vi "DZIELENIE_Z_RESZTA.vi"() -> ()   [LabVIEW 2018]
panel:
  out "reszta":dbl
  out "iloraz":dbl
  in  "dzielnik(ró¿ny od 0)":dbl
  in  "dzielna":dbl
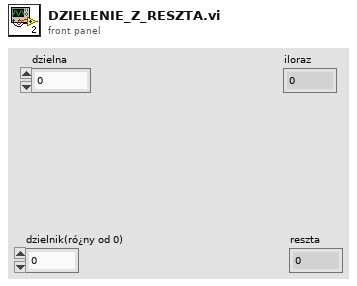
[diagram p1: front panel]
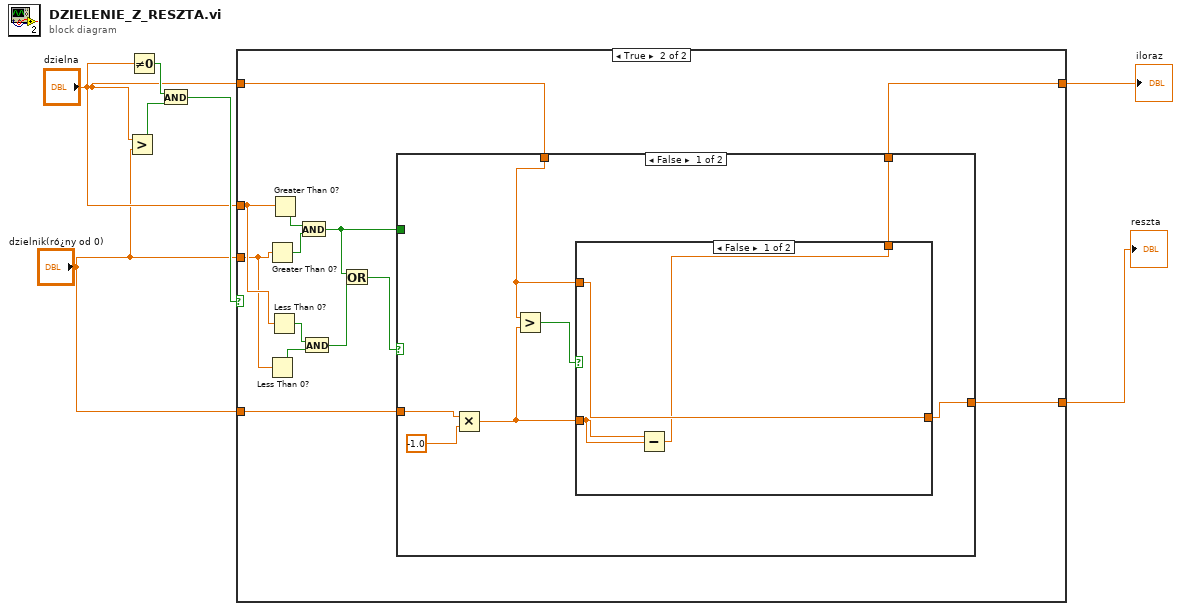
[diagram p0: block diagram]
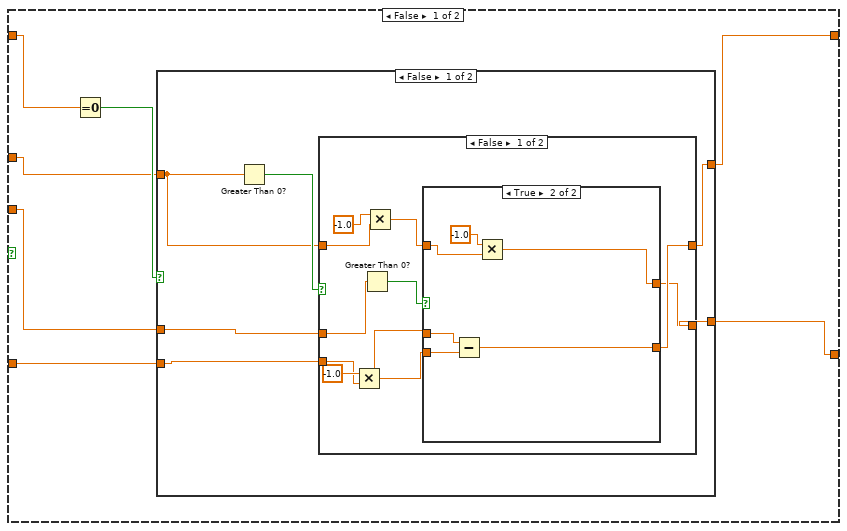
[diagram p2: hidden frame]
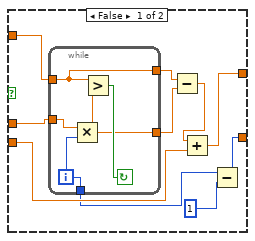
[diagram p3: hidden frame]
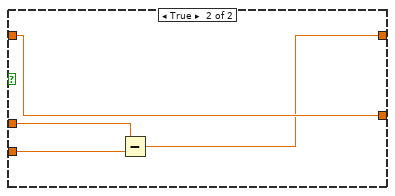
[diagram p4: hidden frame]
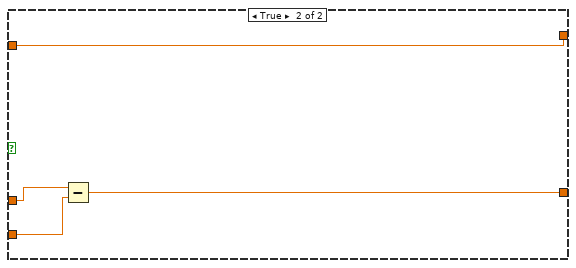
[diagram p5: hidden frame]
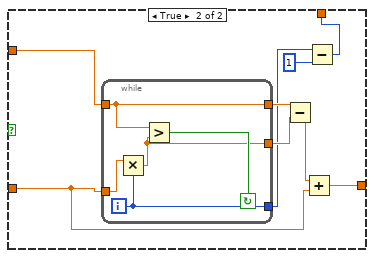
[diagram p6: hidden frame]
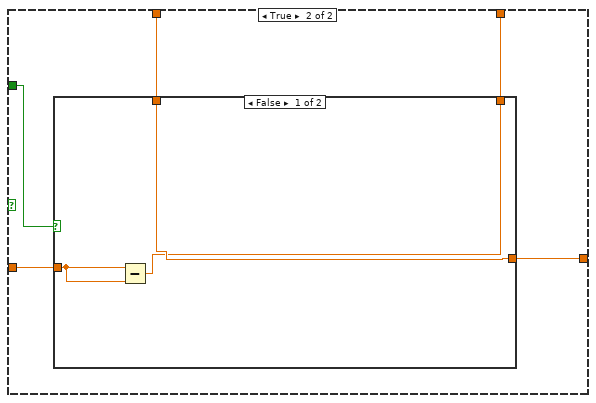
[diagram p7: hidden frame]
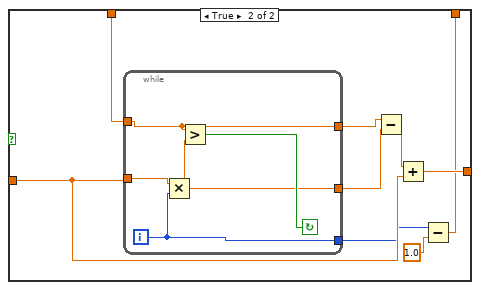
[diagram p8: hidden frame]
diagram:
  n1 = Greater?(x="dzielna", y="dzielnik(ró¿ny od 0)") -> (0:w6:bool)
  n2 = Not Equal To 0?(x="dzielna") -> (x != 0?=w7:bool)
  n3 = And(x=w7, y=w6) -> (x .and. y?=w5:bool)
  n4 = case shown="True" w5 {
    tunnel: "dzielna" -> [w12 w72]
    tunnel: "dzielnik(ró¿ny od 0)" -> [w11 w71]
    tunnel: "dzielna" -> [w14 w63]
    tunnel: "dzielnik(ró¿ny od 0)" -> [w10 w62]
    tunnel: [w9 w61] -> w2
    tunnel: [w8 w60] -> w1
    frame False {
      n5 = Equal To 0?(x=w14) -> (x = 0?=w13:bool)
      n6 = case shown="False" w13 {
        tunnel: w12 -> [w19 w56]
        tunnel: w11 -> [w16 w59]
        tunnel: w10 -> [w15 w58]
        tunnel: [w17 w57] -> w9
        tunnel: [w18 w56] -> w8
        frame False {
          n7 = Greater Than 0?(x=w19) -> (x > 0?=w20:bool)
          n8 = case shown="False" w20 {
            tunnel: w19 -> [w26 w55]
            tunnel: [w28 w52] -> w18
            tunnel: [w27 w55] -> w17
            tunnel: w16 -> [w29 w54]
            tunnel: w15 -> [w22 w53]
            frame False {
              n9 = Multiply(x=-1.0, y=w22) -> (x*y=w21:dbl)
              n10 = Greater Than 0?(x=w29) -> (x > 0?=w30:bool)
              n11 = Multiply(x=-1.0 ("y"), y=w26) -> (x*y=w24:dbl)
              n12 = case shown="True" w30 {
                tunnel: w21 -> [w40 w51]
                tunnel: w21 -> [w38 w50]
                tunnel: [w34 w49] -> w28
                tunnel: w24 -> [w33 w46]
                tunnel: [w37 w47] -> w27
                frame False {
                  n13 = while {
                    tunnel: w33 -> [w43]
                    tunnel: w40 -> [w45]
                    tunnel: [w43] -> w39
                    tunnel: [w42] -> w32
                    tunnel: [w41] -> w36
                    i -> [w41]
                    stop <- w44 continue-if-true
                    n14 = Multiply(x=w45, y=w41) -> (x*y=w42:dbl)
                    n15 = Greater?(x=w43, y=w42) -> (0:w44:bool)
                  }
                  n16 = Subtract(x=w39, y=w32) -> (x-y=w31:dbl)
                  n17 = Add(x=w31, y=w38) -> (x+y=w37:dbl)
                  n18 = Subtract(x=w36, y=1) -> (x-y=w34:i32)
                }
                frame True {
                  n19 = Subtract(x=w51, y=w50) -> (x-y=w49:dbl)
                  n20 = Multiply(x=-1.0 ("x*y"), y=w46) -> (x*y=w47:dbl)
                }
              }
            }
            frame True {
              n21 = Subtract(x=w54, y=w53) -> (x-y=w52:dbl)
            }
          }
        }
        frame True {
          n22 = Subtract(x=w59, y=w58) -> (x-y=w57:dbl)
        }
      }
    }
    frame True {
      n23 = Greater Than 0?(x=w71) -> (x > 0?=w68:bool)
      n24 = Less Than 0?(x=w71) -> (x < 0?=w67:bool)
      n25 = Less Than 0?(x=w72) -> (x < 0?=w69:bool)
      n26 = Greater Than 0?(x=w72) -> (x > 0?=w70:bool)
      n27 = And(x=w70, y=w68) -> (x .and. y?=w64:bool)
      n28 = And(x=w69, y=w67) -> (x .and. y?=w66:bool)
      n29 = Or(x=w64, y=w66) -> (x .or. y?=w65:bool)
      n30 = case shown="False" w65 {
        tunnel: w64 -> [_ w101]
        tunnel: w63 -> [w76 w100]
        tunnel: w62 -> [w79 w99]
        tunnel: [w74 w98] -> w61
        tunnel: [w73 w97] -> w60
        frame False {
          n31 = Multiply(x=w79, y=-1.0 ("x*y")) -> (x*y=w75:dbl)
          n32 = Greater?(x=w76, y=w75) -> (0:w77:bool)
          n33 = case shown="False" w77 {
            tunnel: w76 -> [w82 w91]
            tunnel: w75 -> [w81 w88]
            tunnel: [w82 w86] -> w74
            tunnel: [w80 w85] -> w73
            frame False {
              n34 = Subtract(x=w81, y=w81) -> (x-y=w80:dbl)
            }
            frame True {
              n35 = while {
                tunnel: w91 -> [w94]
                tunnel: w88 -> [w95]
                tunnel: [w94] -> w90
                tunnel: [w93] -> w89
                tunnel: [w92] -> w84
                i -> [w92]
                stop <- w96 continue-if-true
                n36 = Multiply(x=w95, y=w92) -> (x*y=w93:dbl)
                n37 = Greater?(x=w94, y=w93) -> (0:w96:bool)
              }
              n38 = Subtract(x=w90, y=w89) -> (x-y=w87:dbl)
              n39 = Add(x=w87, y=w88) -> (x+y=w86:dbl)
              n40 = Subtract(x=w84, y=1 ("x-y")) -> (x-y=w85:i32)
            }
          }
        }
        frame True {
          n41 = case shown="False" w101 {
            tunnel: w100 -> [w104 w113]
            tunnel: w99 -> [w103 w110]
            tunnel: [w104 w108] -> w98
            tunnel: [w102 w105] -> w97
            frame False {
              n42 = Subtract(x=w103, y=w103) -> (x-y=w102:dbl)
            }
            frame True {
              n43 = while {
                tunnel: w113 -> [w116]
                tunnel: w110 -> [w117]
                tunnel: [w116] -> w112
                tunnel: [w115] -> w111
                tunnel: [w114] -> w106
                i -> [w114]
                stop <- w118 continue-if-true
                n44 = Multiply(x=w117, y=w114) -> (x*y=w115:dbl)
                n45 = Greater?(x=w116, y=w115) -> (0:w118:bool)
              }
              n46 = Subtract(x=w112, y=w111) -> (x-y=w109:dbl)
              n47 = Add(x=w109, y=w110) -> (x+y=w108:dbl)
              n48 = Subtract(x=w106, y=1.0) -> (x-y=w105:dbl)
            }
          }
        }
      }
    }
  }
  "iloraz" <- w1
  "reszta" <- w2
